vi "Nested Class Demo.vi"() -> ()   [LabVIEW 2015]
uses:
  NewBase/NewBase.lvclass
  Nested/Nested.lvclass
  Nested/Nested.lvclass/Nested.ctl
  NewBase/NewBase.lvclass/NewBase.ctl
  Nested/Write Nested value.vi
  NewBase/Write Numeric.vi
  NewBase/Write Nested.vi
panel:
  out "data":refnum<class "NewBase.lvclass">
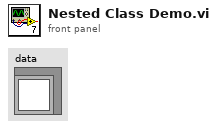
[diagram p1: front panel]
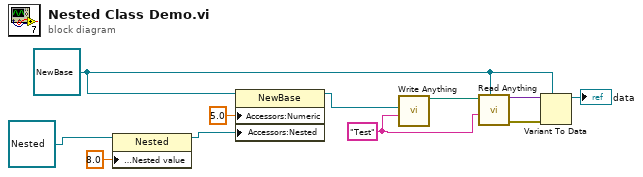
[diagram p0: block diagram]
diagram:
  w6 = "Test" ("Section Name (Name of \"Anything\")")
  w2 = refnum<class "NewBase.lvclass"> refnum ("NewBase")
  n1 = property class="Nested"(reference=refnum<class "Nested.lvclass"> refnum ("Nested"), "Accessors:Nested value"=8.0 ("Nested value")) -> (reference out=w8:refnum<class "Nested.lvclass">)  [unwired: 1 in, 1 out]
  n2 = property class="NewBase"(reference=w2, "Accessors:Numeric"=5.0 ("Numeric"), "Accessors:Nested"=w8) -> (reference out=w7:refnum<class "NewBase.lvclass">)  [unwired: 1 in, 1 out]
  n3 = call "Write Anything.vi"("Section Name (Name of \"Anything\")"=w6, "Anything"=w7) -> ("Path out"=w5:path)  [unwired: 8 in, 1 out]
  n4 = call "Read Anything.vi"("Type of Anything"=w2, "Section Name (Name of \"Type of Anything\")"=w6, "Path (dialog)"=w5) -> ("Error Out"=w4:errorcluster, "Anything"=w3:variant)  [unwired: 6 in, 1 out]
  n5 = Variant To Data(error in=w4, type=w2, Variant=w3) -> (data=→"data":refnum<class "NewBase.lvclass">)  [unwired: 1 out]
